vi "Populate File Review Table.vi"(8 "error in":errorcluster, 11 "Peer Review":refnum<class "Peer Review.lvclass">) -> (0 "error out":errorcluster)   [LabVIEW 2020, in "Peer Review.lvclass"]
uses:
  Peer Review.lvclass
  <vilib>/Utility/miscctls.llb/LVRowAndColumnTypeDef.ctl
  Peer Review.lvclass/Peer Review.ctl
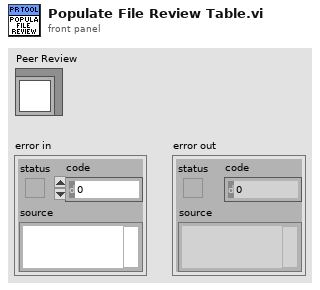
[diagram p1: front panel]
types:
  T1 = typedef "LVRowAndColumnTypeDef.ctl" = cluster{"Row":i32, "Column":i32}
  T2 = typedef "Peer Review.lvclass/File Info.ctl" = cluster{"File ID":i32, "Commit ID":i32, "Reviewed Hash":string, "Relative Path":string, "File Path":path, "File Checksum":string, "State":T3, "FP Changes":i32, "BD Changes":i32, "FP Bounds Error":dbl, "BD Bounds Error":dbl, "Lines Added":i32, "Lines Removed":i32, "Analysis Passes":i32, "Analysis Fails":i32, "Attribute Changes":i32, "Reentrancy Changes":string, "Cyclomatic Complexity":i32, "Node Count":i32, "Revision Number":u32, "LabVIEW Version":string, "Description":string, "Master Path":path, "Master Checksum":string, "VI Type":T4, "LabVIEW File":bool, "Review Complete":bool, "File Ref":refnum<vi>}
  T3 = typedef "Peer Review.lvclass/File State.ctl" = enum16{"Interrogation Needed", "Modified", "Deleted", "Added", "Matches Previous", "No Changes", "Moved"}
  T4 = typedef "Peer Review.lvclass/VI Type.ctl" = enum32{"invalid VI type", "Standard VI", "Control VI", "Global VI", "Polymorphic VI", "Configuration VI", "SubSystem", "Facade VI", "Method VI", "Statechart Diagram VI"}
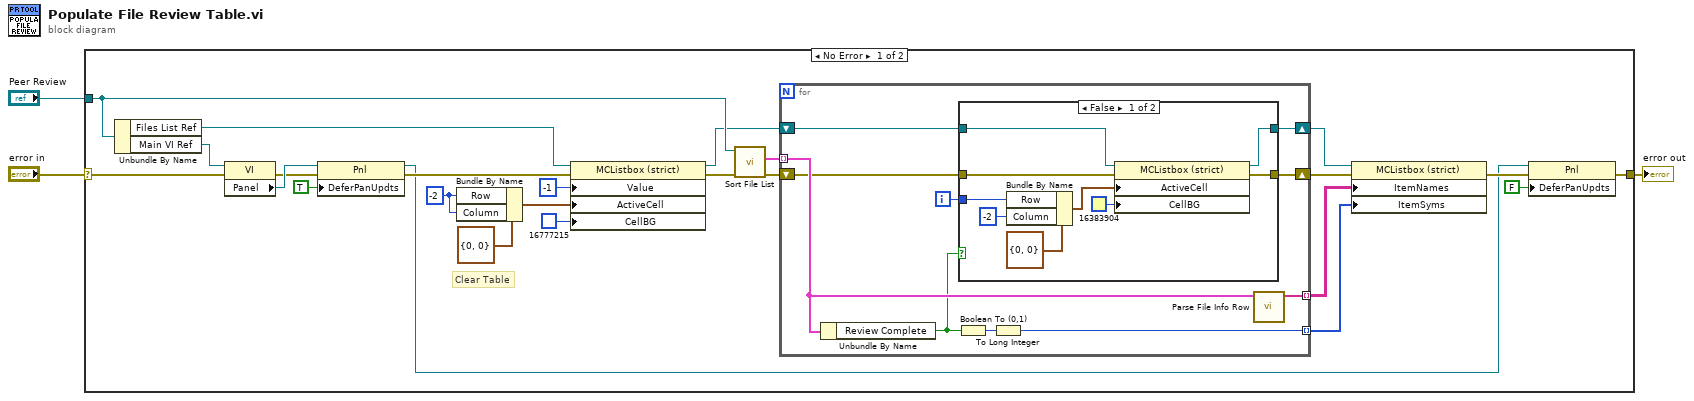
[diagram p0: block diagram]
diagram:
  n1 = case shown="No Error" "error in" {
    selector: "error in" -> [w12 w50]
    tunnel: [w6 w50] -> w2
    tunnel: "Peer Review" -> [w20 _]
    frame No Error {
      w25 = -2 ("Row")
      # "Clear Table"
      n2 = Unbundle By Name(w20) -> ("Files List Ref"=w23:refnum<vi>, "Main VI Ref"=w14:refnum<vi>)
      n3 = property class="VI"(reference=w14, error in=w12) -> (error out=w11:errorcluster, "Panel"=w13:refnum<vi>)  [unwired: 1 out]
      n4 = property class="Pnl"(reference=w13, error in=w11, "DeferPanUpdts"=TRUE ("Defer Panel Updates")) -> (reference out=w5:refnum<vi>, error out=w9:errorcluster)
      n5 = Bundle By Name(cluster=T1 {"Row"=0, "Column"=0} ("Active Cell:Active Cell"), "Row"=w25, "Column"=w25) -> (w26:T1)
      n6 = property class="MCListbox (strict)"(reference=w23, error in=w9, "Value"=-1, "ActiveCell"=w26, "CellBG"=u32 16777215) -> (reference out=w18:refnum<vi>, error out=w22:errorcluster)
      n7 = call "Sort File List.vi"("error in"=w22, "Peer Review"=w20) -> ("error out"=w21:errorcluster, "Sorted File List"=w19:T2[])  [unwired: 8 in]
      n8 = for {
        shift-right: [w35] -> w15
        shift-left: w21 -> [w32]
        tunnel: w19 -> [w37] mode=indexing
        tunnel: [w38] -> w17 mode=indexing
        shift-right: [w33] -> w16
        shift-left: w18 -> [w34]
        tunnel: [w30] -> w4 mode=indexing
        i -> [w36]
        n9 = Unbundle By Name(w37) -> ("Review Complete"=w31:bool)
        n10 = Boolean To (0,1)(Boolean=w31) -> (0, 1=w29:i16)
        n11 = case shown="False" w31 {
          tunnel: w36 -> [w45 _]
          tunnel: w32 -> [w44 w49]
          tunnel: [w41 w49] -> w35
          tunnel: w34 -> [w40 w48]
          tunnel: [w39 w48] -> w33
          frame False {
            n12 = Bundle By Name(cluster=T1 {"Row"=0, "Column"=0} ("Active Cell:Active Cell"), "Row"=w45, "Column"=-2) -> (w43:T1)
            n13 = property on="Property Node" class="MCListbox (strict)"(reference=w40, error in=w44, "ActiveCell"=w43, "CellBG"=u32 16383904) -> (reference out=w39:refnum<vi>, error out=w41:errorcluster)
          }
          frame True {
          }
        }
        n14 = To Long Integer(number=w29) -> (32bit integer=w30:i32)
        n15 = call "Parse File Info Row.vi"("File Info"=w37) -> ("Column Fields"=w38:string[])  [unwired: 10 in]
      }
      n16 = property on="Property Node" class="MCListbox (strict)"(reference=w16, error in=w15, "ItemNames"=w17, "ItemSyms"=w4) -> (error out=w7:errorcluster)  [unwired: 1 out]
      n17 = property class="Pnl"(reference=w5, error in=w7, "DeferPanUpdts"=FALSE ("Defer Panel Updates")) -> (error out=w6:errorcluster)  [unwired: 1 out]
    }
    frame Error {
    }
  }
  "error out" <- w2
